vi "plot2Derror.vi"(10 "length":i32, 11 "2D array":u32[][](array[numeric])) -> (3 "2D Error Bar":refnum<class "2D Plot Datatype.lvclass">[](xcontrol))   [LabVIEW 2018]
uses:
  <vilib>/Math Plots/2D Math Plots/2D Error Bar/2D Error Bar XCtrl/2D Error Bar.xctl
  <vilib>/Math Plots/2D Math Plots/2D Error Bar/2D Error Bar Datatype/Public/Plot Helper (Fixed).vi
  <vilib>/Math Plots/2D Math Plots/2D Error Bar/2D Error Bar Datatype/2D Error Bar Datatype.lvclass
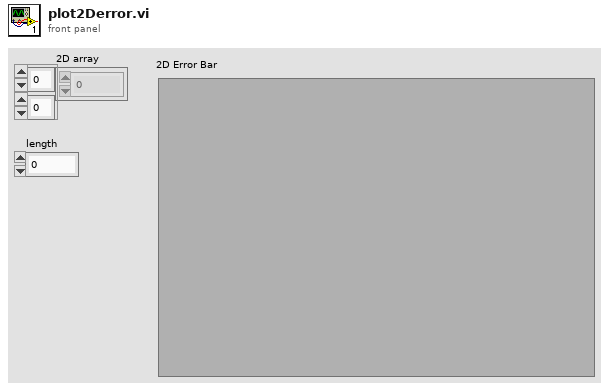
[diagram p1: front panel]
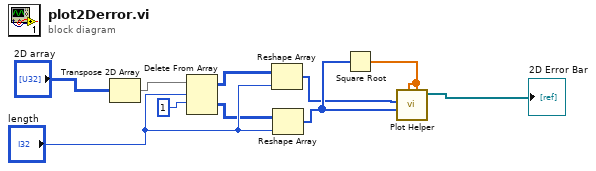
[diagram p0: block diagram]
diagram:
  n1 = Transpose 2D Array(2D array="2D array") -> (transposed array=w3:u32[][])
  n2 = Delete From Array(array=w3, length="length", index (row)=1) -> (deleted portion=w5:u32[][], array with subset deleted=w4:u32[][])  [unwired: 1 in]
  n3 = Reshape Array(w4, "length") -> (w9:u32[])
  n4 = Reshape Array(w5, "length") -> (w10:u32[])
  n5 = Square Root(x=w10) -> (sqrt(x)=w1:dbl[])
  n6 = call-poly <vilib>:"Plot Helper.vi"("error b vector"=w1, "error a vector"=w1, "y vector"=w10, "x vector"=w9) -> ("2D Plot Class Obj Array out"=→"2D Error Bar":refnum<class "2D Plot Datatype.lvclass">[])  [unwired: 2 in, 5 out]
